vi "Test 1.vi"() -> ()   [LabVIEW 2016, in "Drona Path obtn.lvlib"]
uses:
  Drona Path obtn.lvlib
  Typedefs/Test LV2 Enum.ctl
panel:
  out "Drona Path":string
  out "error out":errorcluster
  in  "error in (no error)":errorcluster
  in  "Tab Control":enum32{"Page 1", "Page 2"}(tab)
  in  "Tab Control 2":enum32{"Page 1", "Page 2"}(tab)
  in  "Cluster":cluster{"Numeric":dbl}
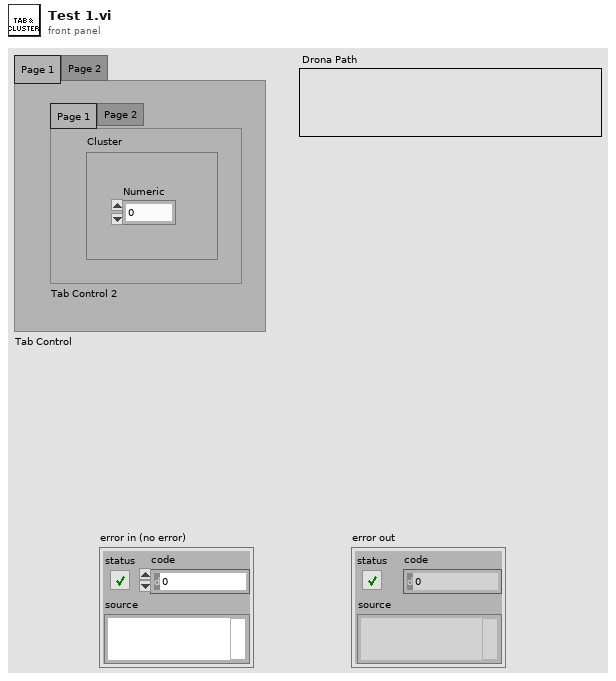
[diagram p1: front panel]
types:
  T1 = typedef "Drona Path obtn.lvlib/Test LV2 Enum.ctl" = enum16{"Initialize", "Write", "Read"}
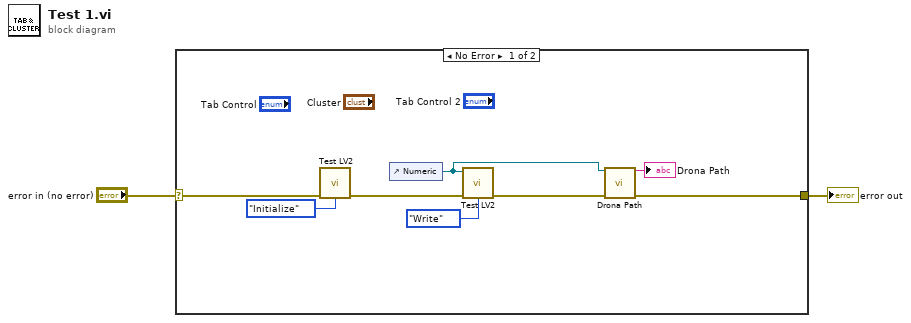
[diagram p0: block diagram]
diagram:
  n1 = case shown="No Error" "error in (no error)" {
    selector: "error in (no error)" -> [w10 w11]
    tunnel: [w5 w11] -> w1
    frame No Error {
      n2 = call "Test LV2.vi"("error in (no error)"=w10, "Operation"=Test_LV2_Enum."Initialize") -> ("error out"=w8:errorcluster)  [unwired: 12 in, 1 out]
      n3 = control-ref of="Numeric"() -> (w4:refnum<vi>)
      n4 = call "Test LV2.vi"("Ref In"=w4, "error in (no error)"=w8, "Operation"=Test_LV2_Enum."Write") -> ("error out"=w6:errorcluster)  [unwired: 11 in, 1 out]
      n5 = call "Drona Path.vi"("Control reference"=w4, "error in (no error)"=w6) -> ("Drona Path"=→"Drona Path":string, "error out"=w5:errorcluster)  [unwired: 12 in]
    }
    frame Error {
    }
  }
  "error out" <- w1
